vi "arrayTo_Graph_asyncCh.vi"(8 "error in (no error)":errorcluster, 10 "Time":dbl[](array[numeric]), 11 "Data":variant[](array[variant])) -> (0 "error out":errorcluster, 3 "DataSet":T1)   [LabVIEW 2020, in "OXYGEN_Datastream.lvlib"]
uses:
  OXYGEN_Datastream.lvlib
  TypeDefs/DataPoint_Variant.ctl
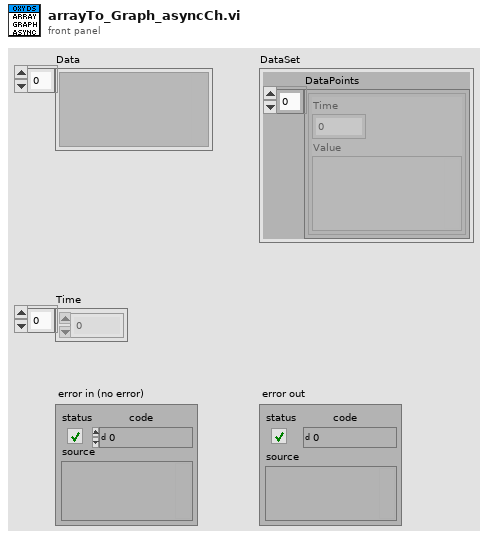
[diagram p1: front panel]
types:
  T1 = typedef "OXYGEN_Datastream.lvlib/DataPoint_Variant.ctl" = cluster{"DataPoints":cluster{"Time":dbl, "Value":variant}[]}
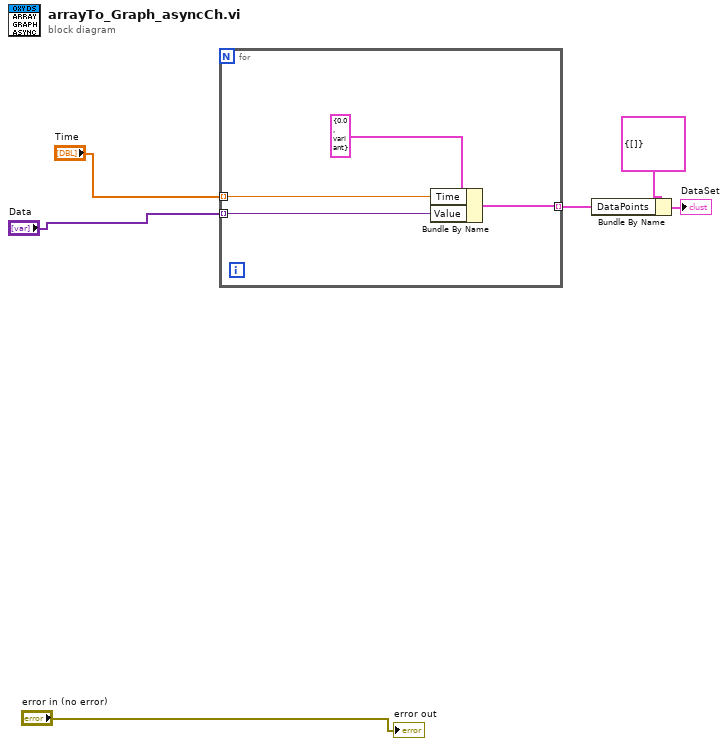
[diagram p0: block diagram]
diagram:
  n1 = for {
    tunnel: "Data" -> [w8] mode=indexing
    tunnel: [w10] -> w5 mode=indexing
    tunnel: "Time" -> [w9] mode=indexing
    n2 = Bundle By Name(cluster=cluster{"Time":dbl, "Value":variant} {"Time"=0.0, "Value"=variant}, "Time"=w9, "Value"=w8) -> (w10:cluster{"Time":dbl, "Value":variant})
  }
  n3 = Bundle By Name(cluster=T1 {"DataPoints"=[]} ("Data"), "DataPoints"=w5) -> (→"DataSet":T1)
  "error out" <- "error in (no error)"
